vi "Stop Core.vi"(10 "final error code":i32, 11 "TCP Connection in":refnum<class "TCP Connection.lvclass">) -> (3 "TCP Connection out":refnum<class "TCP Connection.lvclass">)   [LabVIEW 2012, in "TCP Classes.lvlib" / "TCP Connection.lvclass"]
doc: "(<B>Filename</B>: Actor Framework.lvlib:Actor.lvclass:Stop Core.vi)\n\nDefines what the actor does before it stops. Use the <B>final error code</B> input to determine whether the actor shut down in response to an error.\n\nBy default, this method does nothing. A descendant class may override it to define behavior, such as shutting down any processes the actor initiated in its override of the Actor Core method."
uses:
  TCP Connection.lvclass
  <vilib>/ActorFramework/Actor/Actor.lvclass
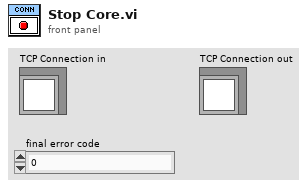
[diagram p1: front panel]
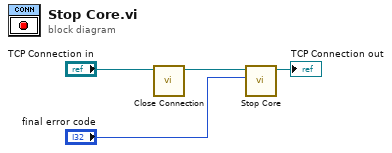
[diagram p0: block diagram]
diagram:
  n1 = call "Close Connection.vi"("TCP Connection in"="TCP Connection in") -> ("TCP Connection out"=w1:refnum<class "TCP Connection.lvclass">)  [unwired: 9 in, 1 out]
  n2 = call-parent "Stop Core.vi"("final error code"="final error code", "Actor in"=w1) -> ("Actor out"=→"TCP Connection out":refnum<class "TCP Connection.lvclass">)  [unwired: 9 in]
